vi "getWeights.vi"(3 "toCopyTo":sgl[][](array[numeric]), 4 "layer":u32, 5 "ptr":i64, 6 "error in":errorcluster) -> (0 "weights":sgl[][](array[numeric]), 1 "ptr Out":i64, 2 "error":errorcluster)   [LabVIEW 2016, in "CNet.lvlib"]
uses:
  CNet.lvlib
  Users/jg754/Documents/Visual Studio 2015/Projects/CLearn/x64/Release/CLearn.dll
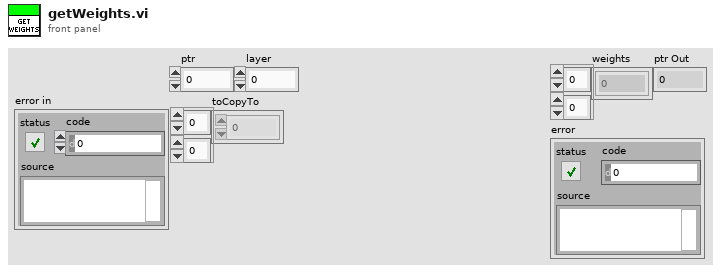
[diagram p1: front panel]
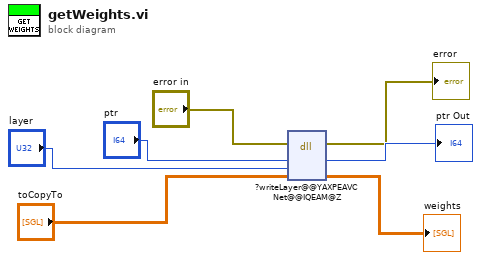
[diagram p0: block diagram]
diagram:
  n1 = dll-call lib="C:/Users/jg754/Documents/Visual Studio 2015/Projects/CLearn/x64/Release/CLearn.dll" fn="?writeLayer@@YAXPEAVCNet@@IQEAM@Z"(error in="error in", "ptr"="ptr", "layer"="layer", "toCopyTo"="toCopyTo") -> (error out=→"error":errorcluster, "ptr"=→"ptr Out":i64, "toCopyTo"=→"weights":sgl[][])  [unwired: 4 in, 1 out]
